vi "Render Model.vi"(4 "3D Picture 2":refnum<vi>, 6 "Reset Camera":bool, 8 "error in (no error)":errorcluster, 9 "Cart X":sgl, 10 "?":T1={"Angle"=0.0, "Lenght"=50.0, "X"=0.0, "Y"=25.0}) -> (0 "error out":errorcluster, 3 "Scene Object Out":refnum<vi>)   [LabVIEW 2017, in "PendulumLoop.lvlib"]
uses:
  PendulumLoop.lvlib
  Render Model.PendulumData.ctl
  <vilib>/Utility/miscctls.llb/LV3DPointTypeDef.ctl
  <vilib>/picture/3D Picture Control/Object/Create Object (name).vi
  <vilib>/picture/3D Picture Control/Object/Add Object (no reference).vi
  <vilib>/picture/3D Picture Control/NI_3D Picture Control.lvlib
panel:
  out "3D Picture":refnum<vi>(3d-picture)
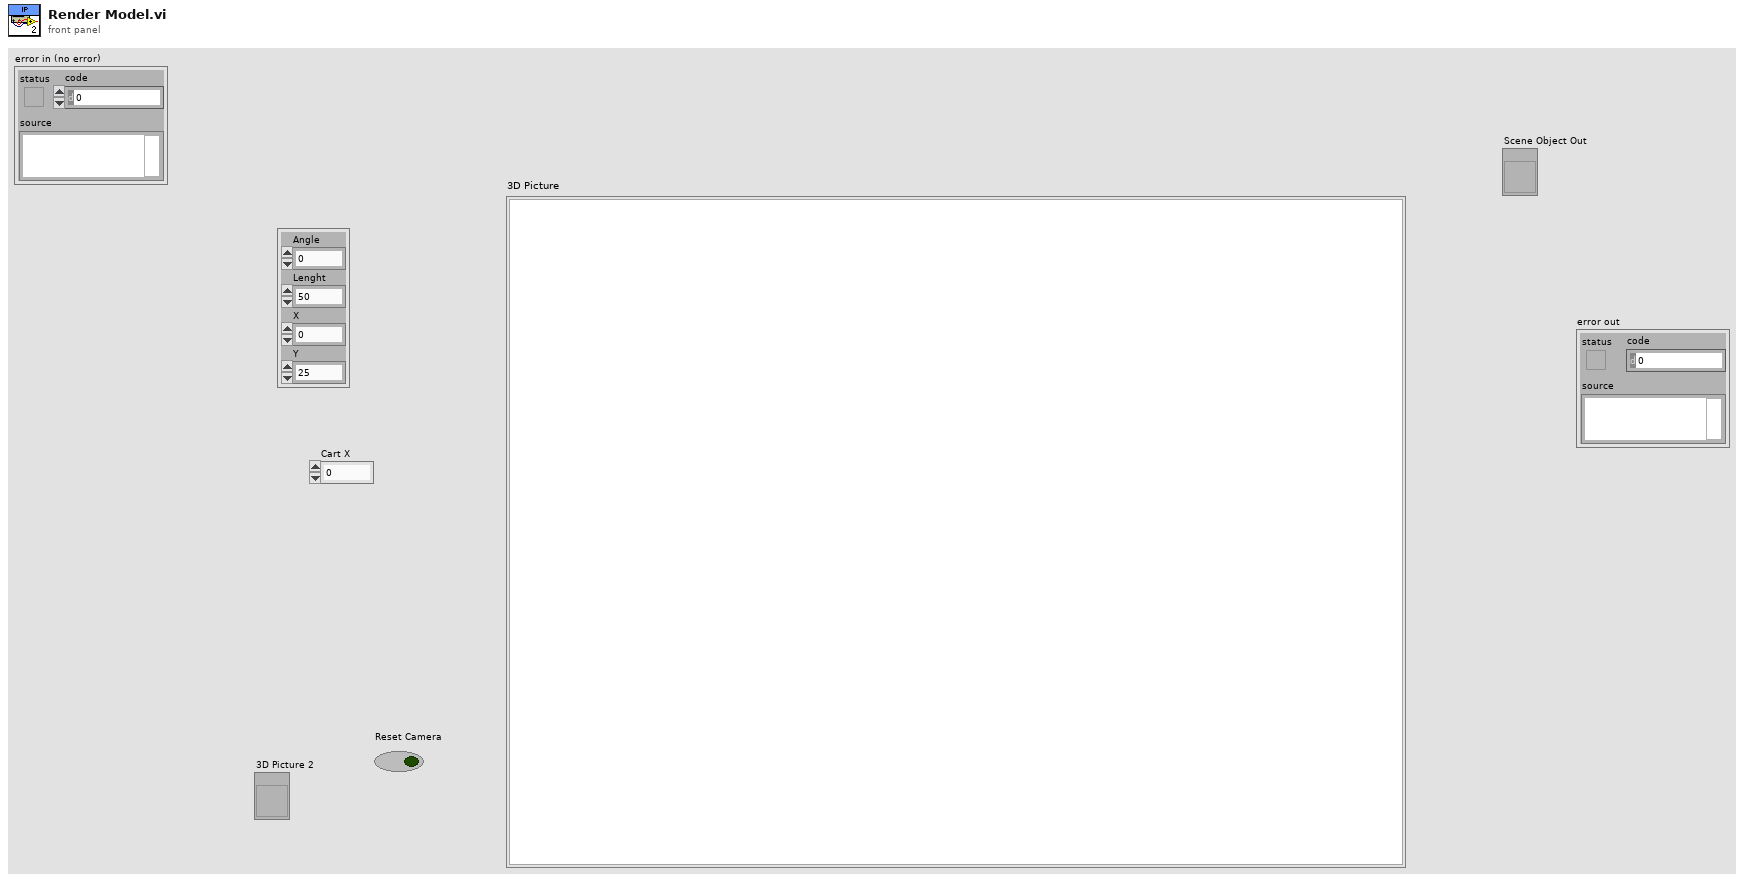
[diagram p1: front panel]
types:
  T1 = typedef "PendulumLoop.lvlib/Render Model.PendulumData.ctl" = cluster{"Angle":sgl, "Lenght":sgl, "X":sgl, "Y":sgl}
  T2 = enum16{"Inherit Value", "Points", "Wireframe", "Polygons"}
  T3 = enum16{"Inherit Value", "Counterclockwise", "Clockwise"}
  T4 = enum16{"Inherit Value", "No Culling", "Cull Back Face", "Cull Front Face", "Cull Both Faces"}
  T5 = typedef "LV3DPointTypeDef.ctl" = cluster{"X":sgl, "Y":sgl, "Z":sgl}
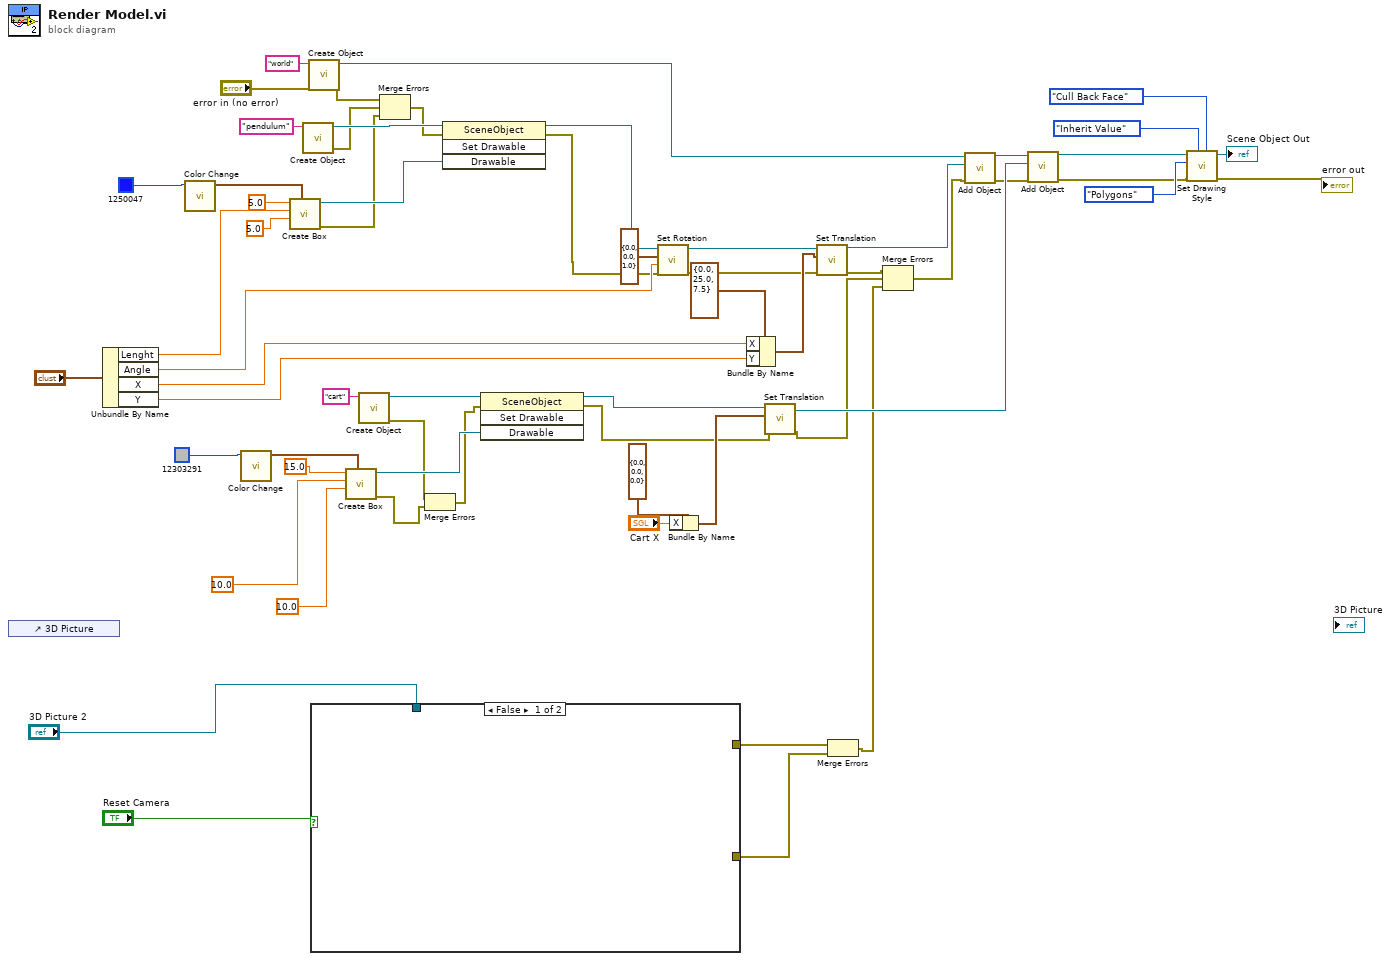
[diagram p0: block diagram]
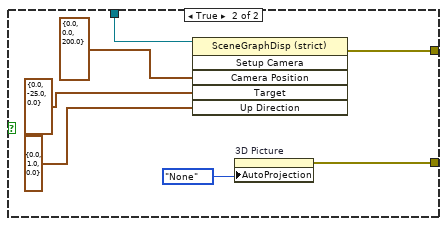
[diagram p2: hidden frame]
diagram:
  n1 = control-ref of="3D Picture"() -> ()  [unwired: 1 out]
  n2 = Unbundle By Name("?") -> ("Lenght"=w26:sgl, "Angle"=w25:sgl, "X"=w24:sgl, "Y"=w23:sgl)
  n3 = call <vilib>:"Color Change.vi"("Color"=u32 1250047 ("Color Box")) -> ("RGBA"=w55:cluster{"R":sgl, "G":sgl, "B":sgl, "A":sgl})  [unwired: 10 in]
  n4 = call <vilib>:"Color Change.vi"("Color"=u32 12303291 ("Color Box")) -> ("RGBA"=w48:cluster{"R":sgl, "G":sgl, "B":sgl, "A":sgl})  [unwired: 10 in]
  n5 = call <vilib>:"Create Box.vi"("Color"=w55, "Length Z"=sgl 5.0, "Length Y"=w26, "Length X"=sgl 5.0) -> ("error out"=w18:errorcluster, "New Box Refnum"=w57:refnum<vi>)  [unwired: 6 in]
  n6 = call-poly <vilib>:"Create Object.vi"("Name"="pendulum") -> ("error out"=w19:errorcluster, "Scene:New Object"=w59:refnum<vi>)  [unwired: 9 in]
  n7 = call-poly <vilib>:"Create Object.vi"("error in (no error)"="error in (no error)", "Name"="world") -> ("error out"=w20:errorcluster, "Scene:New Object"=w58:refnum<vi>)  [unwired: 8 in]
  n8 = case shown="False" "Reset Camera" {
    tunnel: "3D Picture 2" -> [_ w64]
    tunnel: [_ w63] -> w10
    tunnel: [_ w62] -> w9
    frame False {
    }
    frame True {
      n9 = invoke on="Invoke Node" class="SceneGraphDisp (strict)" method="Setup Camera"(reference=w64, "Camera Position"=T5 {"X"=0.0, "Y"=0.0, "Z"=200.0}, "Target"=T5 {"X"=0.0, "Y"=-25.0, "Z"=0.0}, "Up Direction"=T5 {"X"=0.0, "Y"=1.0, "Z"=0.0}) -> (error out=w63:errorcluster)  [unwired: 2 in, 5 out]
      n10 = property on="3D Picture" class="SceneGraphDisp (strict)"("AutoProjection"=enum16{"None", "Perspective", "Orthographic"}."None" ("Automatic Projection Mode")) -> (error out=w62:errorcluster)  [unwired: 2 in, 1 out]
    }
  }
  n11 = call <vilib>:"Create Box.vi"("Color"=w48, "Length Z"=sgl 10.0, "Length Y"=sgl 10.0, "Length X"=sgl 15.0) -> ("error out"=w13:errorcluster, "New Box Refnum"=w46:refnum<vi>)  [unwired: 6 in]
  n12 = call-poly <vilib>:"Create Object.vi"("Name"="cart") -> ("error out"=w14:errorcluster, "Scene:New Object"=w45:refnum<vi>)  [unwired: 9 in]
  n13 = Merge Errors(w20, w19, w18) -> (w17:errorcluster)
  n14 = Merge Errors(w14, w13) -> (w12:errorcluster)
  n15 = invoke class="SceneObject" method="Set Drawable"(reference=w59, error in=w17, "Drawable"=w57) -> (reference out=w41:refnum<vi>, error out=w16:errorcluster)  [unwired: 1 in, 2 out]
  n16 = invoke class="SceneObject" method="Set Drawable"(reference=w45, error in=w12, "Drawable"=w46) -> (reference out=w36:refnum<vi>, error out=w11:errorcluster)  [unwired: 1 in, 2 out]
  n17 = call <vilib>:"Set Rotation.vi"("error in (no error)"=w16, "Angle"=w25, "Axis"=cluster{"X":sgl, "Y":sgl, "Z":sgl} {"X"=0.0, "Y"=0.0, "Z"=1.0}, "Scene Object"=w41) -> ("error out"=w15:errorcluster, "Rotated Scene Object"=w43:refnum<vi>)  [unwired: 6 in]
  n18 = Bundle By Name(cluster=cluster{"X":sgl, "Y":sgl, "Z":sgl} {"X"=0.0, "Y"=0.0, "Z"=0.0} ("Translation 2"), "X"="Cart X") -> (w29:cluster{"X":sgl, "Y":sgl, "Z":sgl})
  n19 = Bundle By Name(cluster=cluster{"X":sgl, "Y":sgl, "Z":sgl} {"X"=0.0, "Y"=25.0, "Z"=7.5} ("Translation"), "X"=w24, "Y"=w23) -> (w31:cluster{"X":sgl, "Y":sgl, "Z":sgl})
  n20 = call <vilib>:"Set Translation.vi"("error in (no error)"=w11, "Translation"=w29, "Scene Object"=w36) -> ("error out"=w7:errorcluster, "Translated Object"=w35:refnum<vi>)  [unwired: 7 in]
  n21 = call <vilib>:"Set Translation.vi"("error in (no error)"=w15, "Translation"=w31, "Scene Object"=w43) -> ("error out"=w8:errorcluster, "Translated Object"=w37:refnum<vi>)  [unwired: 7 in]
  n22 = Merge Errors(w10, w9) -> (w6:errorcluster)
  n23 = Merge Errors(w8, w7, w6) -> (w5:errorcluster)
  n24 = call-poly <vilib>:"Add Object.vi"("error in (no error)"=w5, "New Object In"=w37, "Scene Object In"=w58) -> ("error out"=w4:errorcluster, "Scene Object Out"=w53:refnum<vi>)  [unwired: 7 in]
  n25 = call-poly <vilib>:"Add Object.vi"("error in (no error)"=w4, "New Object In"=w35, "Scene Object In"=w53) -> ("error out"=w3:errorcluster, "Scene Object Out"=w34:refnum<vi>)  [unwired: 7 in]
  n26 = call <vilib>:"Set Drawing Style.vi"("Face Culling Mode"=T4."Cull Back Face", "Frontface Mode"=T3."Inherit Value", "error in (no error)"=w3, "Mode"=T2."Polygons", "Scene Object In"=w34) -> ("error out"=→"error out":errorcluster, "Scene Object Out"=→"Scene Object Out":refnum<vi>)  [unwired: 5 in]
